vi "SensorDataPacketParser.vi"(4 "Message":u8[](array[numeric])) -> (1 "Sensor Data":T1)   [LabVIEW 2014]
uses:
  SensorData.ctl
  navXPacket.ctl
  EncoderPacket.ctl
  PotentiometerPacket.ctl
  distanceSensorPacket.ctl
  switchPacket.ctl
  SensorType.ctl
  SensorStatus.ctl
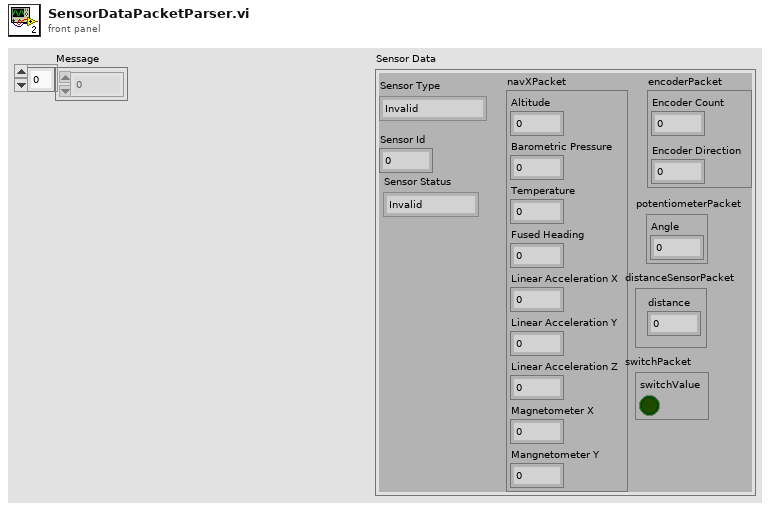
[diagram p1: front panel]
types:
  T1 = typedef "SensorData.ctl" = cluster{"Sensor Id":dbl, "navXPacket":T2, "encoderPacket":T3, "potentiometerPacket":T4, "distanceSensorPacket":T5, "switchPacket":T6, "Sensor Type":T7, "Sensor Status":T8}
  T2 = typedef "navXPacket.ctl" = cluster{"Altitude":dbl, "Barometric Pressure":dbl, "Fused Heading":dbl, "Linear Acceleration Y":dbl, "Linear Acceleration X":dbl, "Temperature":dbl, "Mangnetometer Y":dbl, "Magnetometer X":dbl, "Linear Acceleration Z":dbl}
  T3 = typedef "EncoderPacket.ctl" = cluster{"Encoder Count":dbl, "Encoder Direction":dbl}
  T4 = typedef "PotentiometerPacket.ctl" = cluster{"Angle":dbl}
  T5 = typedef "distanceSensorPacket.ctl" = cluster{"distance":dbl}
  T6 = typedef "switchPacket.ctl" = cluster{"switchValue":bool}
  T7 = typedef "SensorType.ctl" = enum16{"Invalid", "NavX", "Encoder", "Potentiometer", "Distance Sensor", "Switch"}
  T8 = typedef "SensorStatus.ctl" = enum16{"Invalid", "Operational", "Error occurred"}
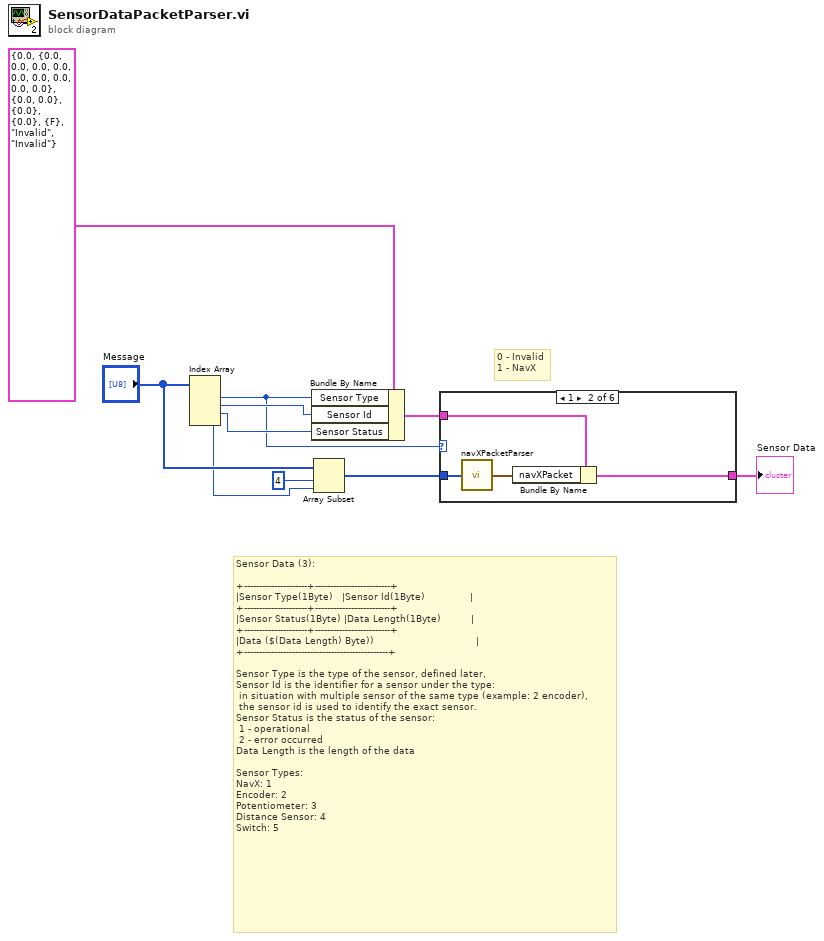
[diagram p0: block diagram]
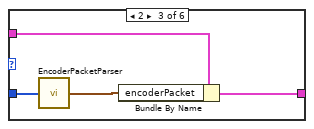
[diagram p3: hidden frame]
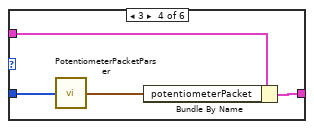
[diagram p4: hidden frame]
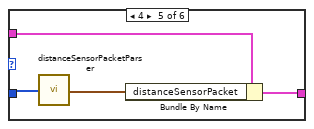
[diagram p5: hidden frame]
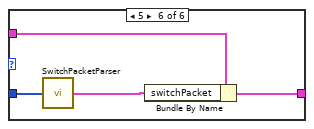
[diagram p6: hidden frame]
diagram:
  # "Sensor Data (3):\n\n+---------------------+-------------------------+\n|Sensor Type(1Byte)   |Sensor Id(1Byte)\t            \t\t|\n+---------------------+-------------------------+\n|Sensor Status(1Byte) |Data Length(1Byte)\t\t        |\n+---------------------+-------------------------+\n|Data ($(Data Length) Byte))\t\t\t\t                             \t|\n+------------------------------------------------+\n\nSensor Type is the type of the sensor, defined later,\nSensor Id is the identifier for a sensor under the type:\n\tin situation with multiple sensor of the same type (example: 2 encoder),\n\tthe sensor id is used to identify the exact sensor.\nSensor Status is the status of the sensor:\n\t1 - operational\n\t2 - error occurred\nData Length is the length of the data\n\nSensor Types:\nNavX: 1\nEncoder: 2\nPotentiometer: 3\nDistance Sensor: 4\nSwitch: 5"
  # "0 - Invalid\n1 - NavX"
  n1 = Index Array(array="Message") -> (element #1=w4:u8, element #2=w9:u8, element #3=w8:u8, element #4=w5:u8)  [unwired: 4 in]
  n2 = Bundle By Name(cluster=T1 {"Sensor Id"=0.0, "navXPacket"={"Altitude"=0.0, "Barometric Pressure"=0.0, "Fused Heading"=0.0, "Linear Acceleration Y"=0.0, "Linear Acceleration X"=0.0, "Temperature"=0.0, "Mangnetometer Y"=0.0, "Magnetometer X"=0.0, "Linear Acceleration Z"=0.0}, "encoderPacket"={"Encoder Count"=0.0, "Encoder Direction"=0.0}, "potentiometerPacket"={"Angle"=0.0}, "distanceSensorPacket"={"distance"=0.0}, "switchPacket"={"switchValue"=FALSE}, "Sensor Type"=enum."Invalid", "Sensor Status"=enum."Invalid"} ("Sensor Data"), "Sensor Type"=w4, "Sensor Id"=w9, "Sensor Status"=w8) -> (w2:T1)
  n3 = Array Subset(array="Message", index=4, length=w5) -> (w3:u8[])
  n4 = case shown="1" w4 {
    tunnel: w3 -> [_ w15 w19 w23 w27 w31]
    tunnel: w2 -> [w11 w14 w17 w21 w26 w30]
    tunnel: [w11 w12 w18 w22 w24 w28] -> w1
    frame 0, Default {
    }
    frame 1 {
      n5 = call "navXPacketParser.vi"("Message"=w15) -> ("navXPacket"=w13:T2)  [unwired: 4 in]
      n6 = Bundle By Name(cluster=w14, "navXPacket"=w13) -> (w12:T1)
    }
    frame 2 {
      n7 = call "EncoderPacketParser.vi"("Message"=w19) -> ("encoderPacket"=w16:T3)  [unwired: 4 in]
      n8 = Bundle By Name(cluster=w17, "encoderPacket"=w16) -> (w18:T1)
    }
    frame 3 {
      n9 = call "PotentiometerPacketParser.vi"("Message"=w23) -> ("Potentiometer Packet Out"=w20:T4)  [unwired: 4 in]
      n10 = Bundle By Name(cluster=w21, "potentiometerPacket"=w20) -> (w22:T1)
    }
    frame 4 {
      n11 = call "distanceSensorPacketParser.vi"("Message"=w27) -> ("distance Sensor Packet Out"=w25:T5)  [unwired: 4 in]
      n12 = Bundle By Name(cluster=w26, "distanceSensorPacket"=w25) -> (w24:T1)
    }
    frame 5 {
      n13 = call "SwitchPacketParser.vi"("Message"=w31) -> ("switch Packet Out"=w29:T6)  [unwired: 4 in]
      n14 = Bundle By Name(cluster=w30, "switchPacket"=w29) -> (w28:T1)
    }
  }
  "Sensor Data" <- w1
